vi "#87_MAV_MSG_POSITION_TARGET_GLOBAL_INT_DECODE.vi"(11 "mavlink_payload":u8[](array[numeric])) -> (3 "POSITION_TARGET_GLOBAL_INT":T1)   [LabVIEW 2023]
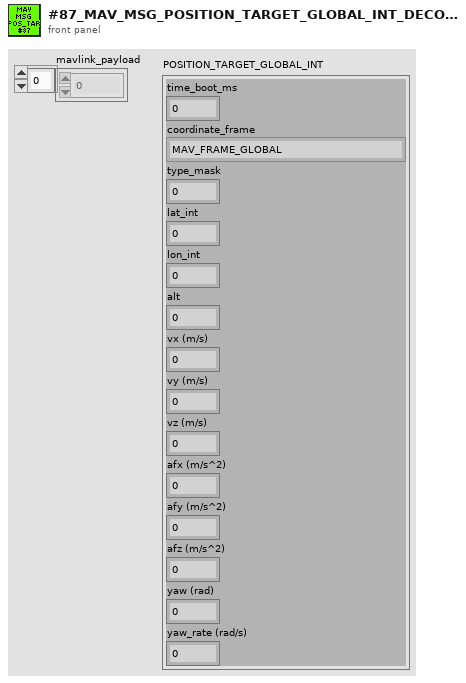
[diagram p1: front panel]
types:
  T1 = cluster{"time_boot_ms":u32, "coordinate_frame":enum8{"MAV_FRAME_GLOBAL", "MAV_FRAME_LOCAL_NED", "MAV_FRAME_MISSION", "MAV_FRAME_GLOBAL_RELATIVE_ALT", "MAV_FRAME_LOCAL_ENU", "MAV_FRAME_GLOBAL_INT", "MAV_FRAME_GLOBAL_RELATIVE_ALT_INT", "MAV_FRAME_LOCAL_OFFSET_NED", "MAV_FRAME_BODY_NED", "MAV_FRAME_BODY_OFFSET_NED", "MAV_FRAME_GLOBAL_TERRAIN_ALT", "MAV_FRAME_GLOBAL_TERRAIN_ALT_INT", "MAV_FRAME_BODY_FRD", "MAV_FRAME_RESERVED_13", "MAV_FRAME_RESERVED_14", "MAV_FRAME_RESERVED_15", "MAV_FRAME_RESERVED_16", "MAV_FRAME_RESERVED_17", "MAV_FRAME_RESERVED_18", "MAV_FRAME_RESERVED_19", "MAV_FRAME_LOCAL_FRD", "MAV_FRAME_LOCAL_FLU"}, "type_mask":u16, "lat_int":i32, "lon_int":i32, "alt":sgl, "vx (m/s)":sgl, "vy (m/s)":sgl, "vz (m/s)":sgl, "afx (m/s^2)":sgl, "afy (m/s^2)":sgl, "afz (m/s^2)":sgl, "yaw (rad)":sgl, "yaw_rate (rad/s)":sgl}
  T2 = enum8{"MAV_FRAME_GLOBAL", "MAV_FRAME_LOCAL_NED", "MAV_FRAME_MISSION", "MAV_FRAME_GLOBAL_RELATIVE_ALT", "MAV_FRAME_LOCAL_ENU", "MAV_FRAME_GLOBAL_INT", "MAV_FRAME_GLOBAL_RELATIVE_ALT_INT", "MAV_FRAME_LOCAL_OFFSET_NED", "MAV_FRAME_BODY_NED", "MAV_FRAME_BODY_OFFSET_NED", "MAV_FRAME_GLOBAL_TERRAIN_ALT", "MAV_FRAME_GLOBAL_TERRAIN_ALT_INT", "MAV_FRAME_BODY_FRD", "MAV_FRAME_RESERVED_13", "MAV_FRAME_RESERVED_14", "MAV_FRAME_RESERVED_15", "MAV_FRAME_RESERVED_16", "MAV_FRAME_RESERVED_17", "MAV_FRAME_RESERVED_18", "MAV_FRAME_RESERVED_19", "MAV_FRAME_LOCAL_FRD", "MAV_FRAME_LOCAL_FLU"}
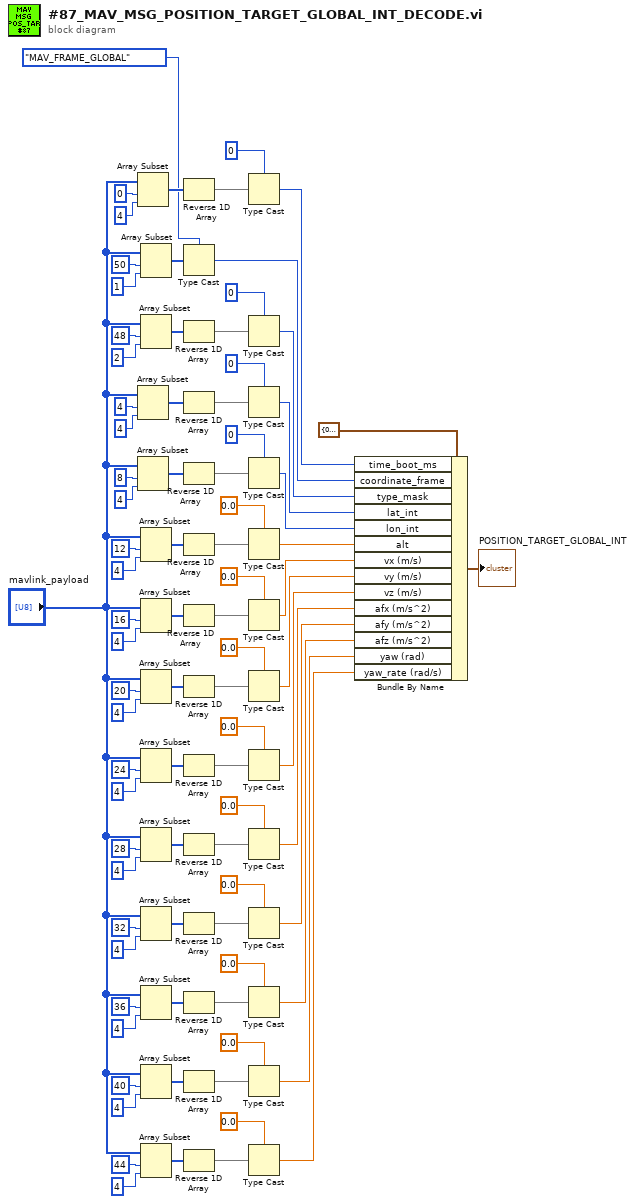
[diagram p0: block diagram]
diagram:
  n1 = Array Subset(array="mavlink_payload", index=0 ("Index"), length=4) -> (w83:u8[])
  n2 = Array Subset(array="mavlink_payload", index=4 ("Index"), length=4) -> (w66:u8[])
  n3 = Array Subset(array="mavlink_payload", index=8 ("Index"), length=4) -> (w60:u8[])
  n4 = Array Subset(array="mavlink_payload", index=50 ("Index"), length=1) -> (w76:u8[])
  n5 = Array Subset(array="mavlink_payload", index=48 ("Index"), length=2) -> (w73:u8[])
  n6 = Array Subset(array="mavlink_payload", index=12 ("Index"), length=4) -> (w54:u8[])
  n7 = Array Subset(array="mavlink_payload", index=16 ("Index"), length=4) -> (w48:u8[])
  n8 = Array Subset(array="mavlink_payload", index=20 ("Index"), length=4) -> (w42:u8[])
  n9 = Array Subset(array="mavlink_payload", index=24 ("Index"), length=4) -> (w36:u8[])
  n10 = Array Subset(array="mavlink_payload", index=28 ("Index"), length=4) -> (w30:u8[])
  n11 = Array Subset(array="mavlink_payload", index=32 ("Index"), length=4) -> (w24:u8[])
  n12 = Array Subset(array="mavlink_payload", index=36 ("Index"), length=4) -> (w18:u8[])
  n13 = Array Subset(array="mavlink_payload", index=40 ("Index"), length=4) -> (w12:u8[])
  n14 = Array Subset(array="mavlink_payload", index=44 ("Index"), length=4) -> (w6:u8[])
  n15 = Reverse 1D Array(array=w83) -> (reversed array=w82:u8[])
  n16 = Type Cast(type=T2."MAV_FRAME_GLOBAL" ("coordinate_frame"), x=w76) -> (*(type *) &x=w75:T2)
  n17 = Reverse 1D Array(array=w73) -> (reversed array=w72:u8[])
  n18 = Reverse 1D Array(array=w66) -> (reversed array=w65:u8[])
  n19 = Reverse 1D Array(array=w60) -> (reversed array=w59:u8[])
  n20 = Reverse 1D Array(array=w54) -> (reversed array=w53:u8[])
  n21 = Reverse 1D Array(array=w48) -> (reversed array=w47:u8[])
  n22 = Reverse 1D Array(array=w42) -> (reversed array=w41:u8[])
  n23 = Reverse 1D Array(array=w36) -> (reversed array=w35:u8[])
  n24 = Reverse 1D Array(array=w30) -> (reversed array=w29:u8[])
  n25 = Reverse 1D Array(array=w24) -> (reversed array=w23:u8[])
  n26 = Reverse 1D Array(array=w18) -> (reversed array=w17:u8[])
  n27 = Reverse 1D Array(array=w12) -> (reversed array=w11:u8[])
  n28 = Reverse 1D Array(array=w6) -> (reversed array=w5:u8[])
  n29 = Type Cast(type=u32 0 ("Index"), x=w82) -> (*(type *) &x=w79:u32)
  n30 = Type Cast(type=u16 0 ("Index"), x=w72) -> (*(type *) &x=w69:u16)
  n31 = Type Cast(type=0 ("Index"), x=w65) -> (*(type *) &x=w62:i32)
  n32 = Type Cast(type=0 ("Index"), x=w59) -> (*(type *) &x=w56:i32)
  n33 = Type Cast(type=sgl 0.0 ("Index"), x=w53) -> (*(type *) &x=w50:sgl)
  n34 = Type Cast(type=sgl 0.0 ("Index"), x=w47) -> (*(type *) &x=w44:sgl)
  n35 = Type Cast(type=sgl 0.0 ("Index"), x=w41) -> (*(type *) &x=w38:sgl)
  n36 = Type Cast(type=sgl 0.0 ("Index"), x=w35) -> (*(type *) &x=w32:sgl)
  n37 = Type Cast(type=sgl 0.0 ("Index"), x=w29) -> (*(type *) &x=w26:sgl)
  n38 = Type Cast(type=sgl 0.0 ("Index"), x=w23) -> (*(type *) &x=w20:sgl)
  n39 = Type Cast(type=sgl 0.0 ("Index"), x=w17) -> (*(type *) &x=w14:sgl)
  n40 = Type Cast(type=sgl 0.0 ("Index"), x=w11) -> (*(type *) &x=w8:sgl)
  n41 = Type Cast(type=sgl 0.0 ("Index"), x=w5) -> (*(type *) &x=w1:sgl)
  n42 = Bundle By Name(cluster=T1 {"time_boot_ms"=0, "coordinate_frame"=enum."MAV_FRAME_GLOBAL", "type_mask"=0, "lat_int"=0, "lon_int"=0, "alt"=0.0, "vx (m/s)"=0.0, "vy (m/s)"=0.0, "vz (m/s)"=0.0, "afx (m/s^2)"=0.0, "afy (m/s^2)"=0.0, "afz (m/s^2)"=0.0, "yaw (rad)"=0.0, "yaw_rate (rad/s)"=0.0} ("POSITION_TARGET_GLOBAL_INT"), "time_boot_ms"=w79, "coordinate_frame"=w75, "type_mask"=w69, "lat_int"=w62, "lon_int"=w56, "alt"=w50, "vx (m/s)"=w44, "vy (m/s)"=w38, "vz (m/s)"=w32, "afx (m/s^2)"=w26, "afy (m/s^2)"=w20, "afz (m/s^2)"=w14, "yaw (rad)"=w8, "yaw_rate (rad/s)"=w1) -> (→"POSITION_TARGET_GLOBAL_INT":T1)
